vi "Module Data Acquisition Loop - FCXF.vi"(7 "Sampling Period (S)":dbl=0.05 caption="采样周期（秒）", 8 "error in (no error)":errorcluster caption="错误输入（无错误）", 11 "Message Queues":T1 caption="消息队列") -> (0 "error out":errorcluster caption="错误输出")   [LabVIEW 2015]
uses:
  Support VIs/Message Queue/All Real-Time Message Queues.ctl
  Support VIs/Message Queue/Message Cluster.ctl
  <vilib>/Platform/TimedLoop/XDataNode/timing_clust.ctl
  <vilib>/Platform/TimedLoop/XDataNode/nitl_modes.ctl
  <vilib>/Platform/TimedLoop/XDataNode/wakeup.ctl
  Globals/Global - Monitoring Variables.vi
  <vilib>/Platform/TimedLoop/XDataNode/loadnilvce.vi
  Globals/Global - All RT Loop Stop.vi
  <vilib>/Platform/TimedLoop/XDataNode/XDataNode.xnode
  <vilib>/Platform/TimedLoop/XDataNode/XDNodeRunTimeDep.lvlib
  Support VIs/Message Queue/Message Queue.lvlib
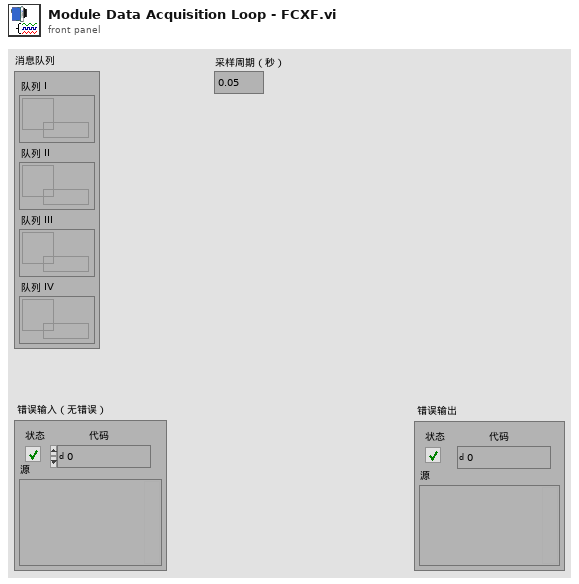
[diagram p1: front panel]
types:
  T1 = typedef "Message Queue.lvlib/All Real-Time Message Queues.ctl" = cluster{"Queue I":refnum<queue>, "Queue II":refnum<queue>, "Queue III":refnum<queue>, "Queue IV":refnum<queue>}
  T2 = typedef "XDNodeRunTimeDep.lvlib/timing_clust.ctl" = cluster{"Expected End [f-1]":u64, "Actual End [f-1]":u64, "Finished Late? [f-1]":bool, "Expected End [i-1]":u64, "Actual End [i-1]":u64, "Finished Late? [i-1]":bool, "Expected Start [i]":u64, "Actual Start [i]":u64, "Expected Start [f]":u64, "Actual Start [f]":u64, "Source Name":string, "Structure Name":string, "Period":i64, "Deadline":i64, "Offset":i64, "Start":i64, "Priority":i32, "Timeout":i32, "Mode":T3, "Wakeup Reason":T4, "Error":errorcluster, "Source Type":string, "Secondary Source Type":string, "Global End Time":u64, "Global Start Time":u64, "Frame Duration":u64, "Iteration Duration":u64, "Assigned CPU":i32, "I/O Scan Engine Mode":u32}
  T3 = typedef "XDNodeRunTimeDep.lvlib/nitl_modes.ctl" = enum32{"No Change", "Process missed periods, maintain original phase", "Discard missed periods, maintain original phase", "Process missed periods, ignore original phase", "Discard missed periods, ignore original phase"}
  T4 = typedef "XDNodeRunTimeDep.lvlib/wakeup.ctl" = enum32{"Normal", "Aborted", "Asynchronous wakeup", "Timing source error", "Timed loop error", "Timeout"}
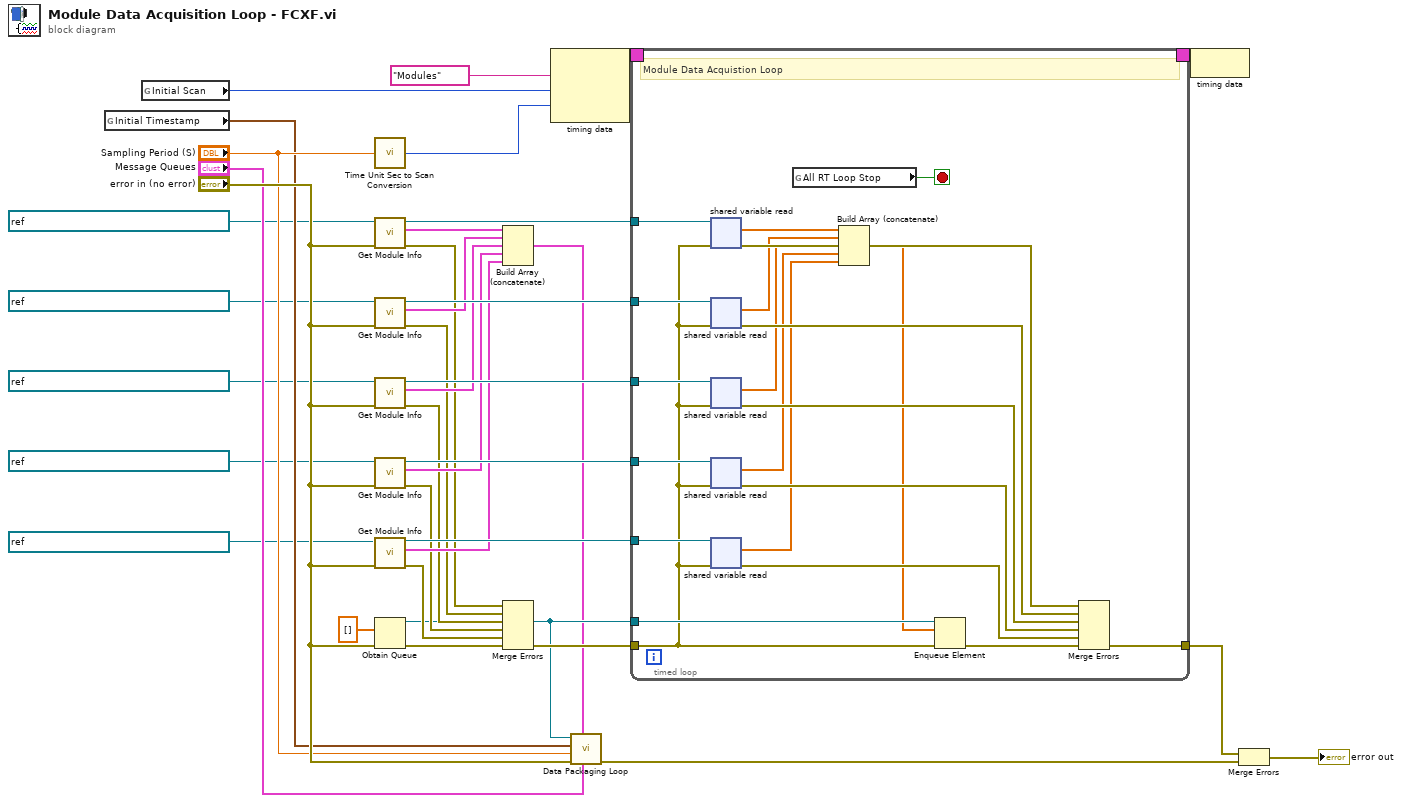
[diagram p0: block diagram]
diagram:
  n1 = global read "Global - Monitoring Variables.vi" "Initial Timestamp"() -> (w6:timestamp)
  n2 = global read "Global - Monitoring Variables.vi" "Initial Scan"() -> (w14:i64)
  n3 = call "Time Unit Sec to Scan Conversion.vi"("time duration (s)"="Sampling Period (S)") -> ("time duration (scan)"=w13:i64)
  n4 = call "Get Module Info.vi"("IO Container"=refnum<k21> "ni.var.io://ni-crio-9036-fcxf/Mod1" ("9239引用句柄"), "error in (no error)"="error in (no error)") -> ("IO Container(dup)"=w32:refnum<k21>, "channel info array"=w23:cluster{"Module":string, "Channel":string}[], "error out"=w22:errorcluster)  [unwired: 6 in]
  n5 = call "Get Module Info.vi"("IO Container"=refnum<k21> "ni.var.io://ni-crio-9036-fcxf/Mod2" ("9219引用句柄"), "error in (no error)"="error in (no error)") -> ("IO Container(dup)"=w31:refnum<k21>, "channel info array"=w24:cluster{"Module":string, "Channel":string}[], "error out"=w21:errorcluster)  [unwired: 6 in]
  n6 = call "Get Module Info.vi"("IO Container"=refnum<k21> "ni.var.io://ni-crio-9036-fcxf/Mod4" ("9219引用句柄"), "error in (no error)"="error in (no error)") -> ("IO Container(dup)"=w30:refnum<k21>, "channel info array"=w25:cluster{"Module":string, "Channel":string}[], "error out"=w20:errorcluster)  [unwired: 6 in]
  n7 = call "Get Module Info.vi"("IO Container"=refnum<k21> "ni.var.io://ni-crio-9036-fcxf/Mod6" ("9219引用句柄"), "error in (no error)"="error in (no error)") -> ("IO Container(dup)"=w29:refnum<k21>, "channel info array"=w26:cluster{"Module":string, "Channel":string}[], "error out"=w19:errorcluster)  [unwired: 6 in]
  n8 = call "Get Module Info.vi"("IO Container"=refnum<k21> "ni.var.io://ni-crio-9036-fcxf/Mod8" ("9219引用句柄"), "error in (no error)"="error in (no error)") -> ("IO Container(dup)"=w28:refnum<k21>, "channel info array"=w27:cluster{"Module":string, "Channel":string}[], "error out"=w18:errorcluster)  [unwired: 6 in]
  n9 = Obtain Queue(element data type=dbl[] [] ("数据类型"), error in (no error)="error in (no error)") -> (queue out=w11:refnum<queue>, error out=w17:errorcluster)  [unwired: 3 in, 1 out]
  n10 = Build Array (concatenate)(w23, w24, w25, w26, w27) -> (w10:cluster{"Module":string, "Channel":string}[])
  n11 = Merge Errors(w22, w21, w20, w19, w18, w17) -> (w16:errorcluster)
  n12 = node-c288("Modules" ("结构名称"), w14, w13) -> (w37:T2)
  n13 = call "Data Packaging Loop.vi"("Message Queues"="Message Queues", "channel info array"=w10, "error in (no error)"="error in (no error)", "sampling period (s)"="Sampling Period (S)", "timestamp"=w6, "data queue"=w11) -> ("error out"=w12:errorcluster)  [unwired: 5 in]
  n14 = timed-loop {
    timing: w37 -> [_]
    timing-out: [_] -> w36
    tunnel: w11 -> [w57]
    tunnel: [w38] -> w33
    tunnel: w32 -> [w45]
    tunnel: w31 -> [w44]
    tunnel: w30 -> [w43]
    tunnel: w29 -> [w42]
    tunnel: w28 -> [w41]
    tunnel: w16 -> [w40]
    stop <- w58 stop-if-true
    # "Module Data Acquistion Loop"
    n15 = shared-variable-read(w45, w40) -> (w52:errorcluster, w51:dbl[])  [unwired: 1 out]
    n16 = shared-variable-read(w44, w40) -> (w53:errorcluster, w50:dbl[])  [unwired: 1 out]
    n17 = shared-variable-read(w43, w40) -> (w54:errorcluster, w49:dbl[])  [unwired: 1 out]
    n18 = shared-variable-read(w42, w40) -> (w55:errorcluster, w48:dbl[])  [unwired: 1 out]
    n19 = shared-variable-read(w41, w40) -> (w56:errorcluster, w47:dbl[])  [unwired: 1 out]
    n20 = global read "Global - All RT Loop Stop.vi" "All RT Loop Stop"() -> (w58:bool)
    n21 = Build Array (concatenate)(w51, w50, w49, w48, w47) -> (w46:dbl[])
    n22 = Enqueue Element(queue=w57, element=w46, error in (no error)=w40) -> (error out=w39:errorcluster)  [unwired: 1 in, 2 out]
    n23 = Merge Errors(w52, w53, w54, w55, w56, w39) -> (w38:errorcluster)
  }
  n24 = node-c288(w36) -> ()
  n25 = Merge Errors(w33, w12) -> (→"error out":errorcluster)
